vi "niDTS WLAN Tx Test Close.vi"(0 "Dummy Test Handle in":T1, 11 "error in (no error)":errorcluster) -> (15 "error out":errorcluster)   [LabVIEW 2014, in "niDTS WLAN.lvlib"]
uses:
  niDTS WLAN.lvlib
  Includes/niDTS WLAN Tx Test INC Handle.ctl
  Objects/BASE_class/niDTS WLAN Tx Test.lvclass
  Framework/Session/Includes/niDTS Session INC Force Destroy.ctl
  Framework/niDTS Framework.lvlib
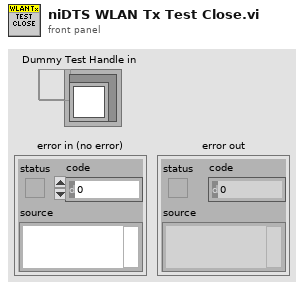
[diagram p1: front panel]
types:
  T1 = typedef "niDTS WLAN.lvlib/niDTS WLAN Tx Test INC Handle.ctl" = refnum<data-value>
  T2 = typedef "niDTS Framework.lvlib/niDTS Session INC Force Destroy.ctl" = bool
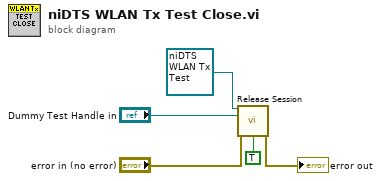
[diagram p0: block diagram]
diagram:
  n1 = call-dynamic "Release Session.vi"("OBJ - Session in"=refnum<class "niDTS WLAN Tx Test.lvclass"> refnum ("Dummy Test.lvlib:Dummy Test.lvclass"), "Session Handle in"="Dummy Test Handle in", "error in (no error)"="error in (no error)", "Force Destroy? (F)"=T2 TRUE) -> ("error out"=→"error out":errorcluster)  [unwired: 10 in, 1 out]
